vi "Update Impedance.vi"(8 "EEG Data":cluster{"WiBCI16T Data out":T1, "En MAP":u16} {"WiBCI16T Data out"."Reg Map"."ADS2" format="%x"; "WiBCI16T Data out"."Reg Map"."ADS1" format="%x"}, 9 "Numeric":u8, 11 "Data Cluster in":T4) -> (3 "Data Cluster out":T4)   [LabVIEW 2019, in "CML UI.lvlib"]
uses:
  CML UI.lvlib
  Module Data--cluster.ctl
  Acquisition State.ctl
  Measurement UI Displays.ctl
  Acquisition/WiBCI16T_Data.ctl
  Acquisition/WiBCI16T_Status.ctl
  Acquisition/Reg_Map.ctl
  Acquisition/Acquisition.lvlib
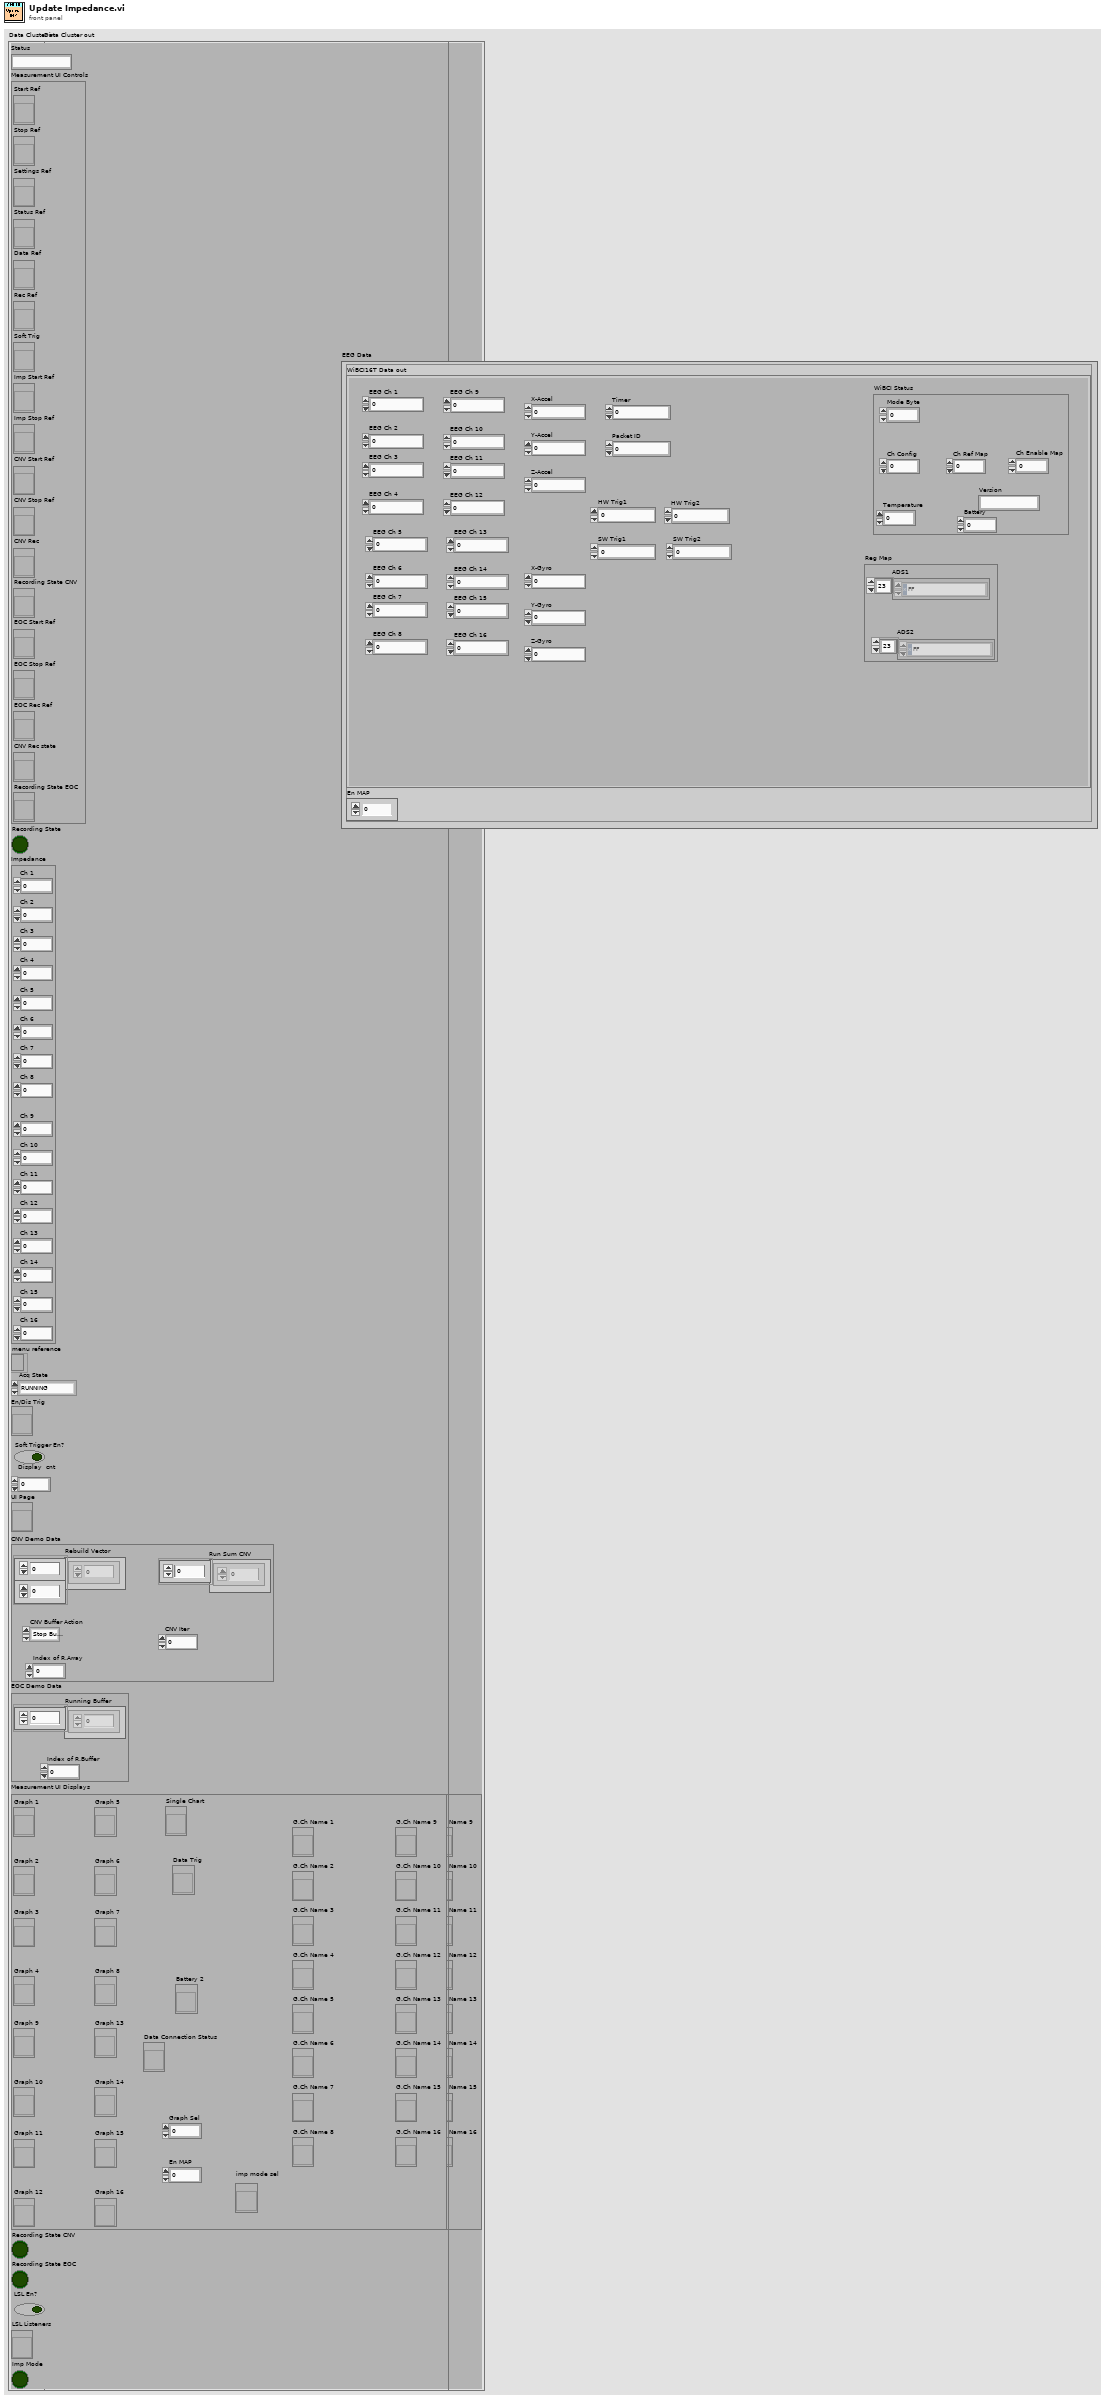
[diagram p1: front panel]
types:
  T1 = typedef "Acquisition.lvlib/WiBCI16T_Data.ctl" = cluster{"EEG Ch 1":dbl, "EEG Ch 2":dbl, "EEG Ch 3":dbl, "EEG Ch 4":dbl, "EEG Ch 5":dbl, "EEG Ch 6":dbl, "EEG Ch 7":dbl, "EEG Ch 8":dbl, "EEG Ch 9":dbl, "EEG Ch 10":dbl, "EEG Ch 11":dbl, "EEG Ch 12":dbl, "EEG Ch 13":dbl, "EEG Ch 14":dbl, "EEG Ch 15":dbl, "EEG Ch 16":dbl, "X-Accel":i16, "Y-Accel":i16, "Z-Accel":i16, "X-Gyro":i16, "Y-Gyro":i16, "Z-Gyro":i16, "Timer":u32, "Packet ID":u32, "HW Trig1":u8, "SW Trig1":i8, "HW Trig2":u8, "SW Trig2":i8, "WiBCI Status":T2, "Reg Map":T3}
  T2 = typedef "Acquisition.lvlib/WiBCI16T_Status.ctl" = cluster{"Mode Byte":u8, "Ch Config":u8, "Ch Ref Map":u16, "Ch Enable Map":u16, "Temperature":sgl, "Battery":u8, "Version":string}
  T3 = typedef "Acquisition.lvlib/Reg_Map.ctl" = cluster{"ADS1":u8[], "ADS2":u8[]}
  T4 = typedef "CML UI.lvlib/Module Data--cluster.ctl" = cluster{"Status":string, "Measurement UI Controls":cluster{"Start Ref":refnum<vi>, "Stop Ref":refnum<vi>, "Settings Ref":refnum<vi>, "Status Ref":refnum<vi>, "Data Ref":refnum<vi>, "Rec Ref":refnum<vi>, "Soft Trig":refnum<vi>, "Imp Start Ref":refnum<vi>, "Imp Stop Ref":refnum<vi>, "CNV Start Ref":refnum<vi>, "CNV Stop Ref":refnum<vi>, "CNV Rec":refnum<vi>, "Recording State CNV":refnum<vi>, "EOC Start Ref":refnum<vi>, "EOC Stop Ref":refnum<vi>, "EOC Rec Ref":refnum<vi>, "CNV Rec state":refnum<vi>, "Recording State EOC":refnum<vi>}, "Recording State":bool, "Impedance":cluster{"Ch 1":dbl, "Ch 2":dbl, "Ch 3":dbl, "Ch 4":dbl, "Ch 5":dbl, "Ch 6":dbl, "Ch 7":dbl, "Ch 8":dbl, "Ch 9":dbl, "Ch 10":dbl, "Ch 11":dbl, "Ch 12":dbl, "Ch 13":dbl, "Ch 14":dbl, "Ch 15":dbl, "Ch 16":dbl}, "menu reference ":refnum<k9>, "Acq State":T5, "En/Dis Trig":refnum<vi>, "Soft Trigger En?":bool, "Display  cnt":u8, "UI Page":refnum<vi>, "CNV Demo Data":cluster{"Rebuild Vector":dbl[][], "CNV Buffer Action":enum16{"Stop Buffer Fill", "Start Buffer Fill", "Analyze Buffer"}, "Index of R.Array":u16, "Run Sum CNV":dbl[], "CNV Iter":u16}, "EOC Demo Data":cluster{"Running Buffer":dbl[], "Index of R.Buffer":u8}, "Measurement UI Displays":T6, "Recording State CNV":bool, "Recording State EOC":bool, "LSL En?":bool, "LSL Listeners":refnum<vi>, "Imp Mode":bool}
  T5 = typedef "CML UI.lvlib/Acquisition State.ctl" = enum16{"RUNNING", "IDLE"}
  T6 = typedef "CML UI.lvlib/Measurement UI Displays.ctl" = cluster{"Graph 1":refnum<vi>, "Graph 2":refnum<vi>, "Graph 3":refnum<vi>, "Graph 4":refnum<vi>, "Graph 5":refnum<vi>, "Graph 6":refnum<vi>, "Graph 7":refnum<vi>, "Graph 8":refnum<vi>, "Graph 9":refnum<vi>, "Graph 10":refnum<vi>, "Graph 11":refnum<vi>, "Graph 12":refnum<vi>, "Graph 13":refnum<vi>, "Graph 14":refnum<vi>, "Graph 15":refnum<vi>, "Graph 16":refnum<vi>, "Battery 2":refnum<vi>, "Data Trig":refnum<vi>, "Data Connection Status":refnum<vi>, "Graph Sel":u8, "En MAP":u16, "Single Chart":refnum<vi>, "G.Ch Name 1":refnum<vi>, "G.Ch Name 2":refnum<vi>, "G.Ch Name 3":refnum<vi>, "G.Ch Name 4":refnum<vi>, "G.Ch Name 5":refnum<vi>, "G.Ch Name 6":refnum<vi>, "G.Ch Name 7":refnum<vi>, "G.Ch Name 8":refnum<vi>, "G.Ch Name 9":refnum<vi>, "G.Ch Name 10":refnum<vi>, "G.Ch Name 11":refnum<vi>, "G.Ch Name 12":refnum<vi>, "G.Ch Name 13":refnum<vi>, "G.Ch Name 14":refnum<vi>, "G.Ch Name 15":refnum<vi>, "G.Ch Name 16":refnum<vi>, "imp mode sel":refnum<vi>}
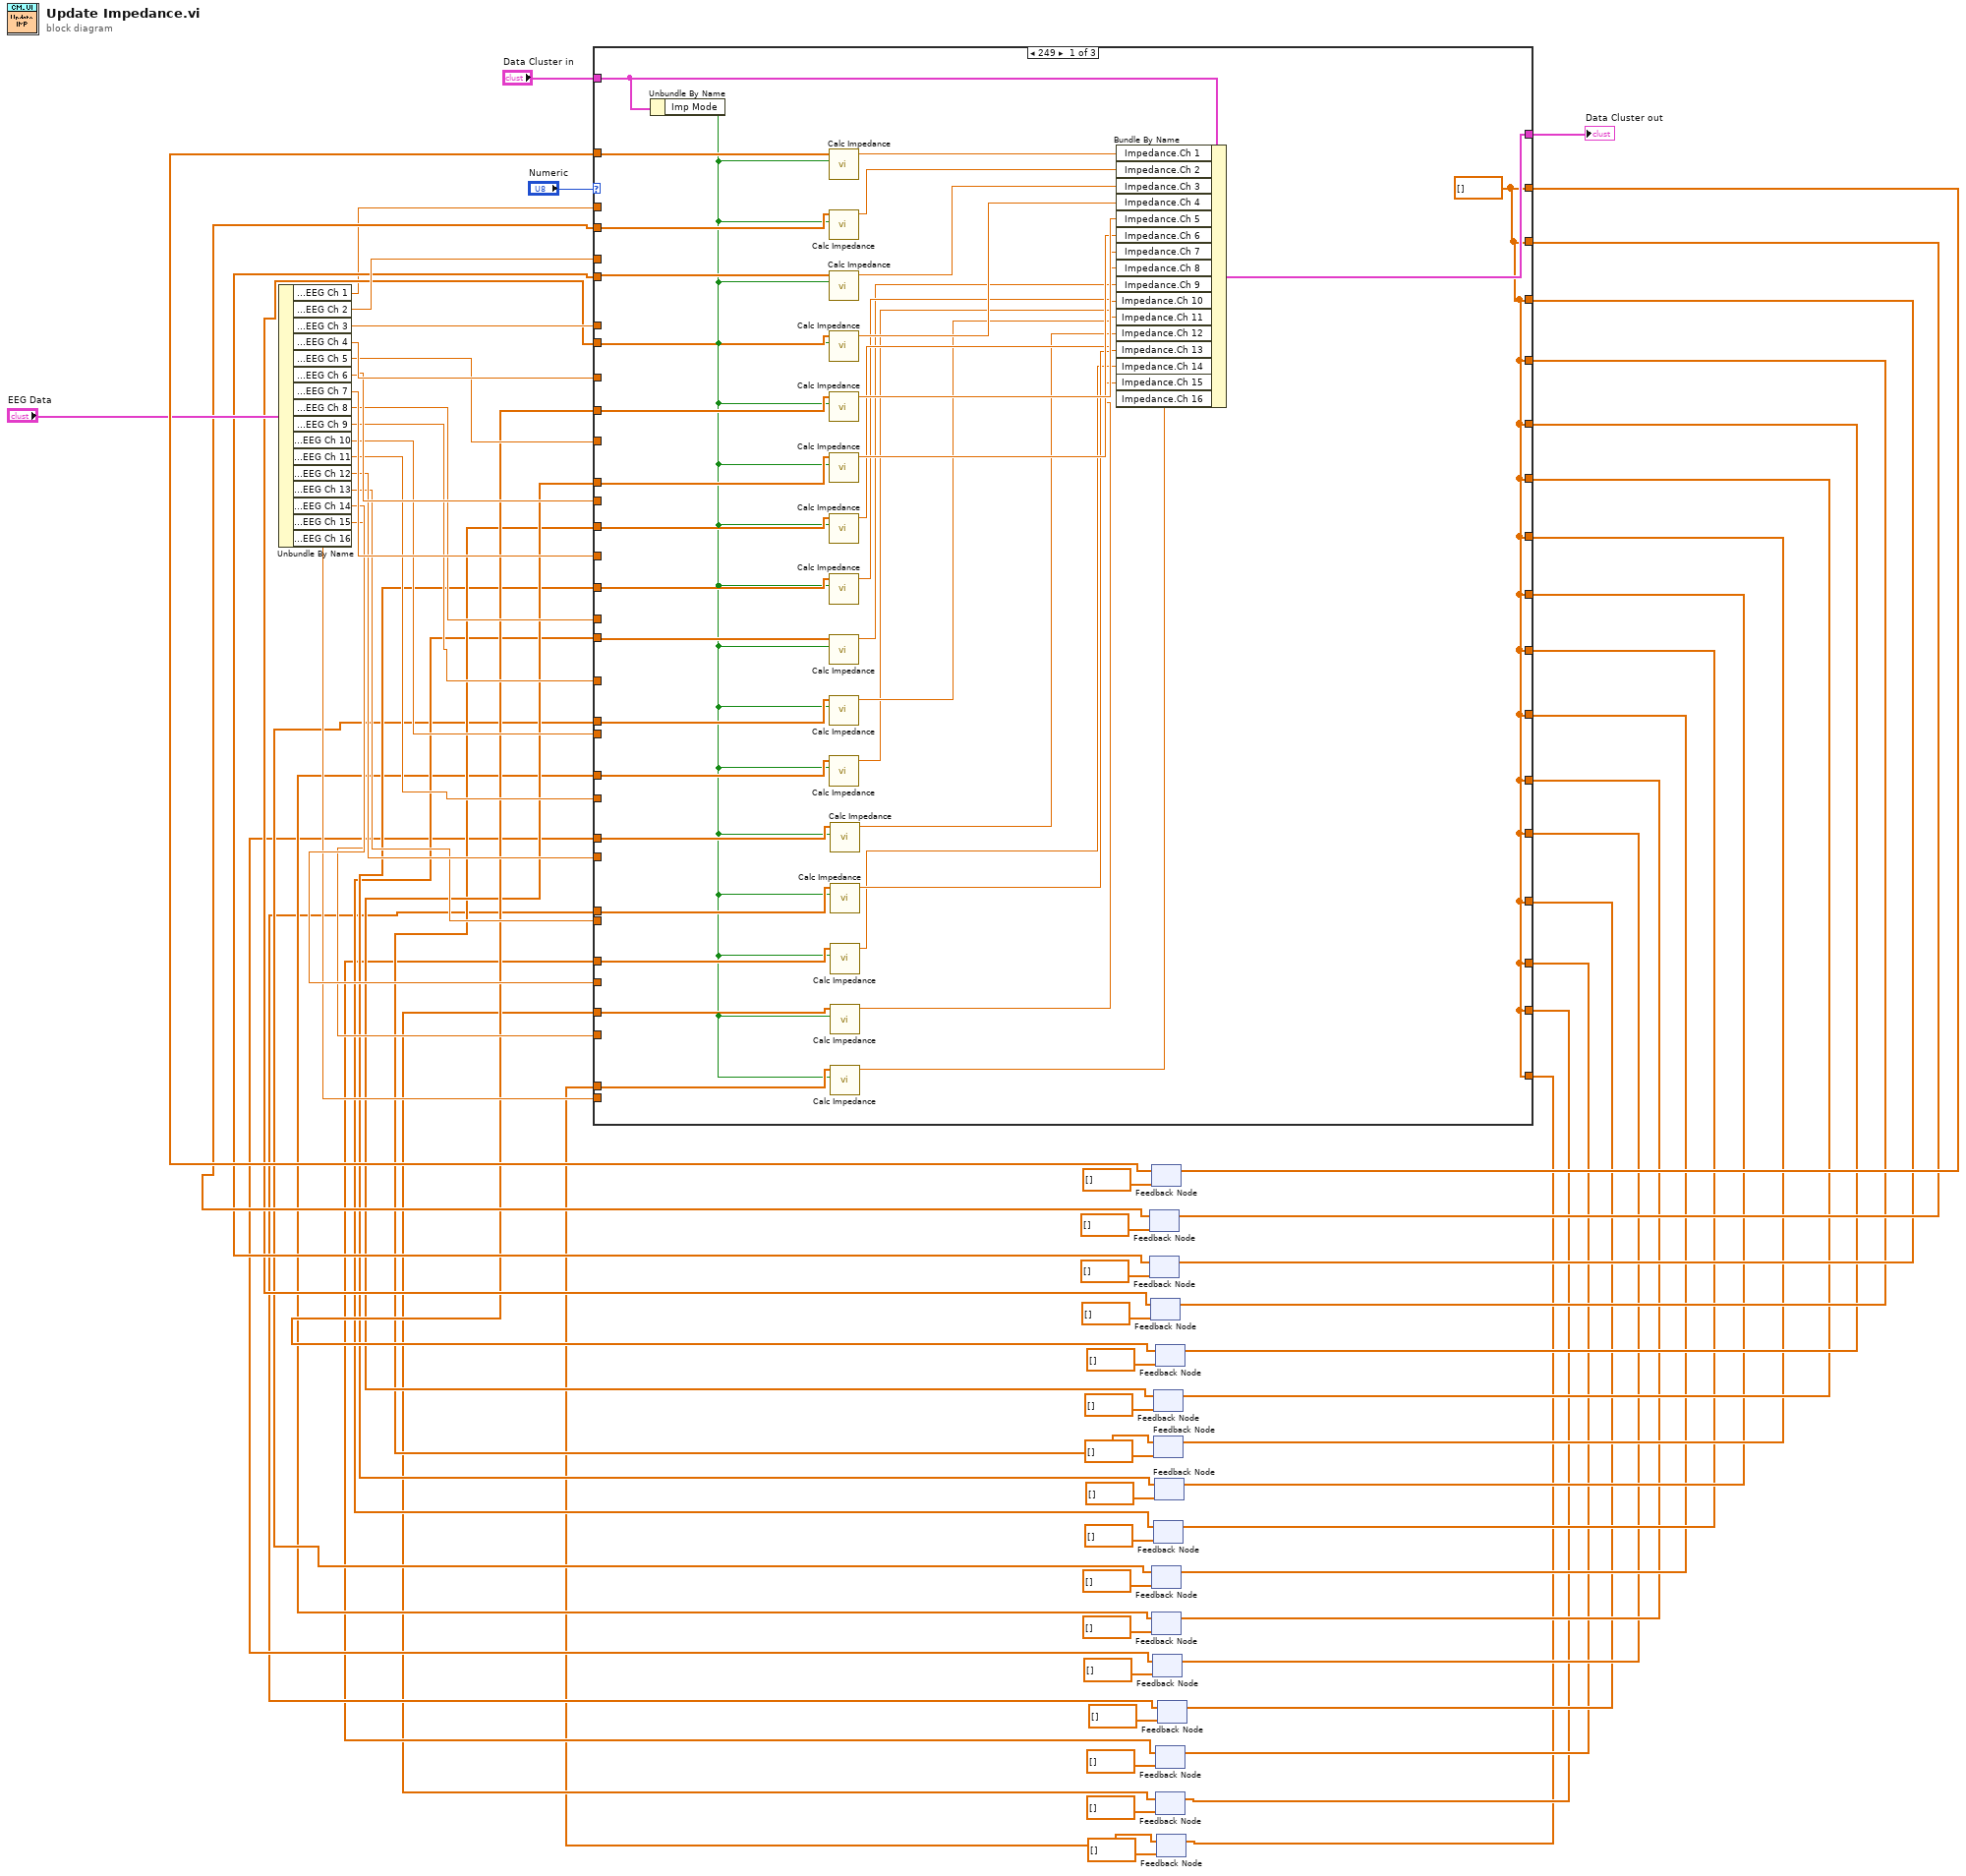
[diagram p0: block diagram]
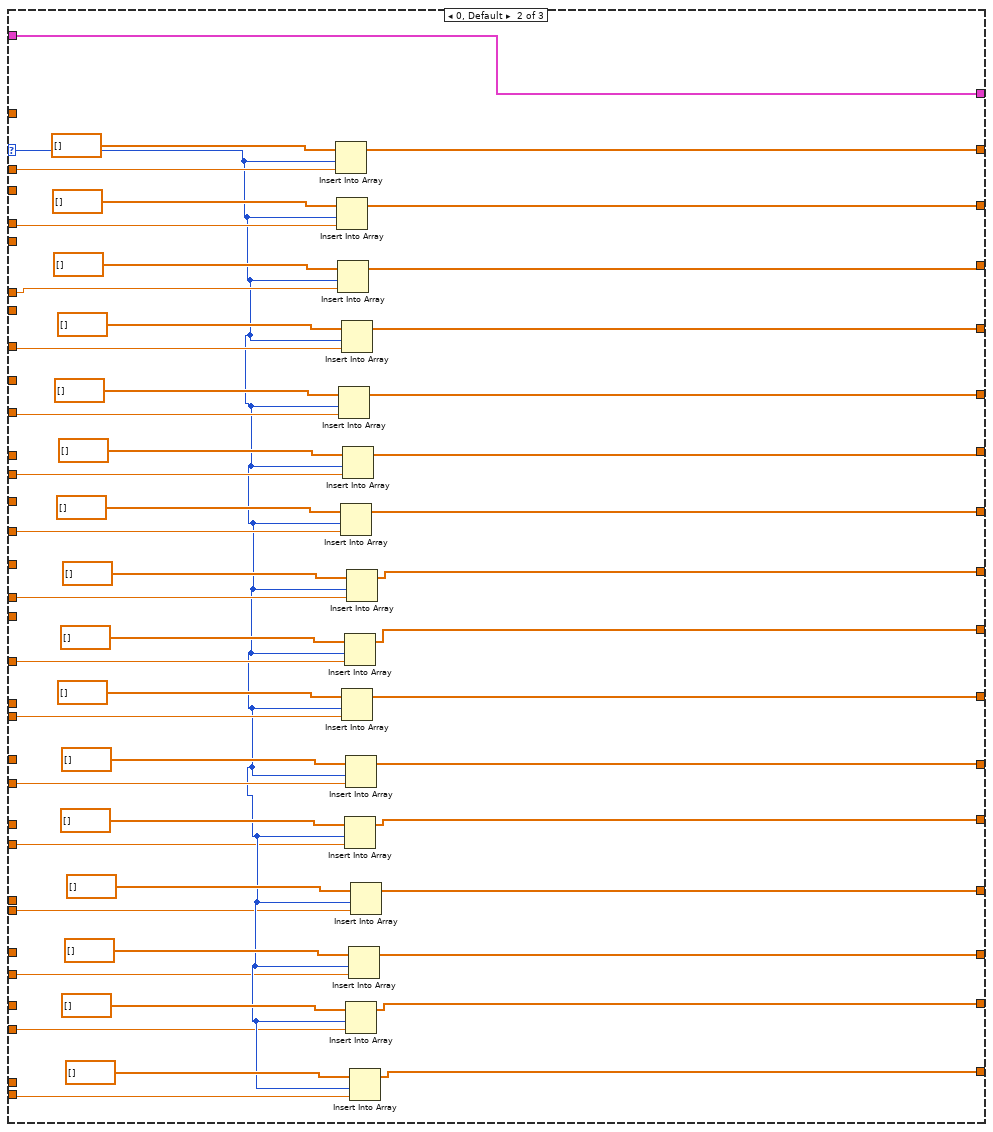
[diagram p2: hidden frame]
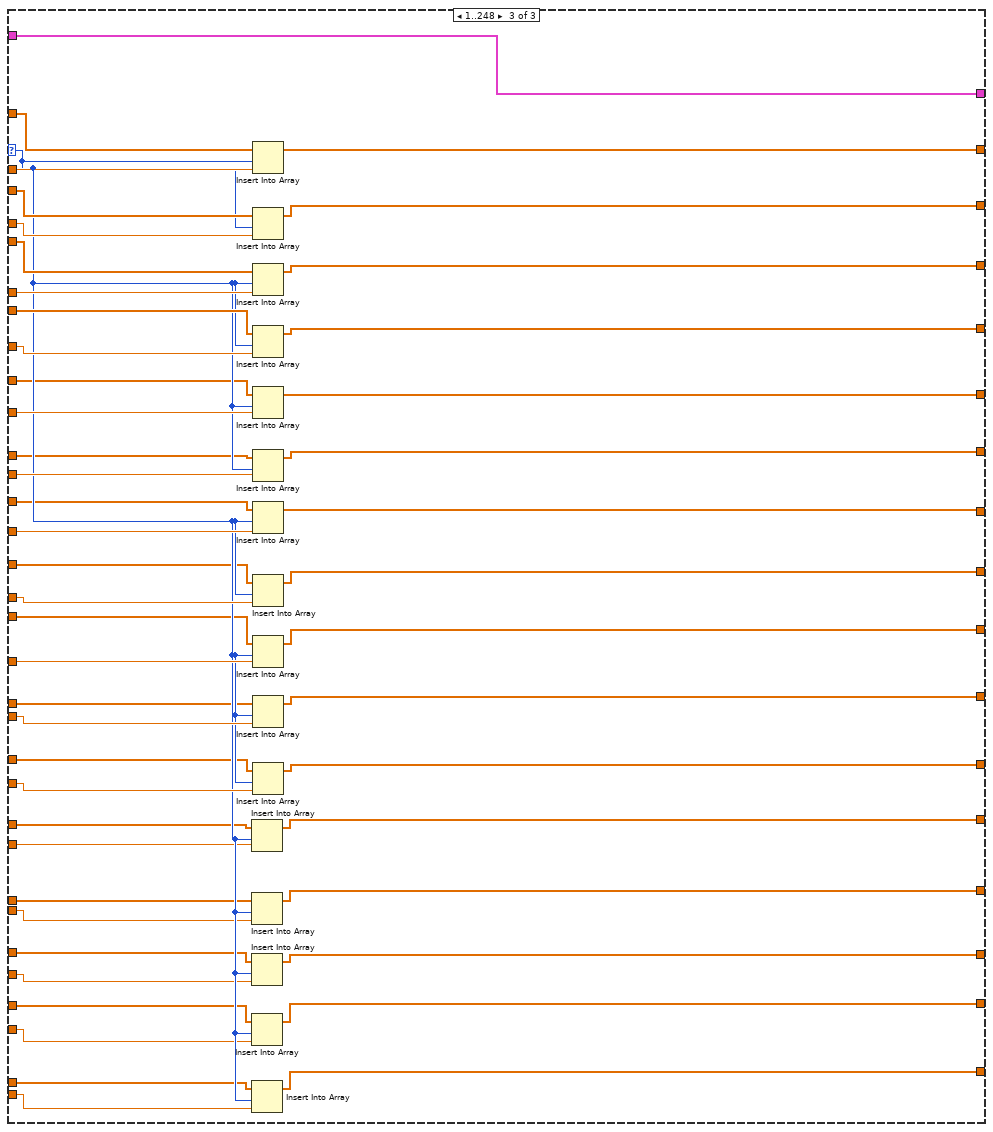
[diagram p3: hidden frame]
diagram:
  n1 = Unbundle By Name("EEG Data") -> ("WiBCI16T Data out.EEG Ch 1"=w1:dbl, "WiBCI16T Data out.EEG Ch 2"=w61:dbl, "WiBCI16T Data out.EEG Ch 3"=w60:dbl, "WiBCI16T Data out.EEG Ch 4"=w59:dbl, "WiBCI16T Data out.EEG Ch 5"=w58:dbl, "WiBCI16T Data out.EEG Ch 6"=w57:dbl, "WiBCI16T Data out.EEG Ch 7"=w56:dbl, "WiBCI16T Data out.EEG Ch 8"=w55:dbl, "WiBCI16T Data out.EEG Ch 9"=w54:dbl, "WiBCI16T Data out.EEG Ch 10"=w53:dbl, "WiBCI16T Data out.EEG Ch 11"=w52:dbl, "WiBCI16T Data out.EEG Ch 12"=w51:dbl, "WiBCI16T Data out.EEG Ch 13"=w50:dbl, "WiBCI16T Data out.EEG Ch 14"=w49:dbl, "WiBCI16T Data out.EEG Ch 15"=w48:dbl, "WiBCI16T Data out.EEG Ch 16"=w47:dbl)
  n2 = feedback #1(dbl[] []) -> (w31:dbl[])
  n3 = feedback #2(dbl[] []) -> (w30:dbl[])
  n4 = feedback #3(dbl[] []) -> (w29:dbl[])
  n5 = feedback #4(dbl[] []) -> (w64:dbl[])
  n6 = feedback #5(dbl[] []) -> (w8:dbl[])
  n7 = feedback #6(dbl[] []) -> (w7:dbl[])
  n8 = feedback #7(dbl[] []) -> (w6:dbl[])
  n9 = feedback #8(dbl[] []) -> (w12:dbl[])
  n10 = feedback #9(dbl[] []) -> (w11:dbl[])
  n11 = feedback #10(dbl[] []) -> (w9:dbl[])
  n12 = feedback #11(dbl[] []) -> (w10:dbl[])
  n13 = feedback #12(dbl[] []) -> (w13:dbl[])
  n14 = feedback #13(dbl[] []) -> (w4:dbl[])
  n15 = feedback #14(dbl[] []) -> (w3:dbl[])
  n16 = feedback #15(dbl[] []) -> (w2:dbl[])
  n17 = feedback #16(dbl[] []) -> (w5:dbl[])
  n18 = case shown="249" "Numeric" {
    selector: "Numeric" -> [_ w125 w177]
    tunnel: [w73 w153 w204] -> w63
    tunnel: w64 -> [w72 _ w202]
    tunnel: w1 -> [_ w152 w203]
    tunnel: "Data Cluster in" -> [w70 w151 w201]
    tunnel: [w103 w151 w201] -> w68
    tunnel: w61 -> [_ w140 w198]
    tunnel: w60 -> [_ w139 w197]
    tunnel: w59 -> [_ w138 w196]
    tunnel: w58 -> [_ w137 w194]
    tunnel: w57 -> [_ w136 w193]
    tunnel: w56 -> [_ w135 w192]
    tunnel: w55 -> [_ w134 w191]
    tunnel: w54 -> [_ w133 w190]
    tunnel: w53 -> [_ w132 w189]
    tunnel: w52 -> [_ w131 w188]
    tunnel: w51 -> [_ w124 w176]
    tunnel: w50 -> [_ w123 w175]
    tunnel: w49 -> [_ w122 w174]
    tunnel: w48 -> [_ w121 w173]
    tunnel: w47 -> [_ w120 w172]
    tunnel: [w73 w119 w187] -> w28
    tunnel: [w73 w118 w186] -> w27
    tunnel: [w73 w117 w185] -> w26
    tunnel: [w73 w116 w184] -> w25
    tunnel: [w73 w115 w183] -> w24
    tunnel: [w73 w114 w182] -> w23
    tunnel: [w73 w113 w181] -> w22
    tunnel: [w73 w112 w180] -> w21
    tunnel: [w73 w111 w179] -> w20
    tunnel: [w73 w110 w178] -> w19
    tunnel: [w73 w109 w171] -> w18
    tunnel: [w73 w108 w170] -> w17
    tunnel: [w73 w107 w169] -> w16
    tunnel: [w73 w106 w168] -> w15
    tunnel: [w73 w105 w167] -> w14
    tunnel: w31 -> [w71 _ w200]
    tunnel: w30 -> [w102 _ w199]
    tunnel: w29 -> [w101 _ w195]
    tunnel: w13 -> [w100 _ w166]
    tunnel: w12 -> [w99 _ w165]
    tunnel: w11 -> [w98 _ w164]
    tunnel: w10 -> [w97 _ w163]
    tunnel: w9 -> [w96 _ w162]
    tunnel: w8 -> [w95 _ w161]
    tunnel: w7 -> [w94 _ w160]
    tunnel: w6 -> [w93 _ w159]
    tunnel: w5 -> [w92 _ w158]
    tunnel: w4 -> [w91 _ w157]
    tunnel: w3 -> [w90 _ w156]
    tunnel: w2 -> [w89 _ w155]
    frame 249 {
      w73 = dbl[] []
      n19 = Unbundle By Name(w70) -> ("Imp Mode"=w69:bool)
      n20 = call "Calc Impedance.vi"("imp mode"=w69, "Array"=w72) -> ("Impedance"=w104:dbl)  [unwired: 9 in]
      n21 = call "Calc Impedance.vi"("imp mode"=w69, "Array"=w71) -> ("Impedance"=w88:dbl)  [unwired: 9 in]
      n22 = call "Calc Impedance.vi"("imp mode"=w69, "Array"=w102) -> ("Impedance"=w87:dbl)  [unwired: 9 in]
      n23 = call "Calc Impedance.vi"("imp mode"=w69, "Array"=w101) -> ("Impedance"=w86:dbl)  [unwired: 9 in]
      n24 = call "Calc Impedance.vi"("imp mode"=w69, "Array"=w100) -> ("Impedance"=w85:dbl)  [unwired: 9 in]
      n25 = call "Calc Impedance.vi"("imp mode"=w69, "Array"=w99) -> ("Impedance"=w84:dbl)  [unwired: 9 in]
      n26 = call "Calc Impedance.vi"("imp mode"=w69, "Array"=w98) -> ("Impedance"=w83:dbl)  [unwired: 9 in]
      n27 = call "Calc Impedance.vi"("imp mode"=w69, "Array"=w97) -> ("Impedance"=w82:dbl)  [unwired: 9 in]
      n28 = call "Calc Impedance.vi"("imp mode"=w69, "Array"=w96) -> ("Impedance"=w81:dbl)  [unwired: 9 in]
      n29 = call "Calc Impedance.vi"("imp mode"=w69, "Array"=w95) -> ("Impedance"=w80:dbl)  [unwired: 9 in]
      n30 = call "Calc Impedance.vi"("imp mode"=w69, "Array"=w94) -> ("Impedance"=w79:dbl)  [unwired: 9 in]
      n31 = call "Calc Impedance.vi"("imp mode"=w69, "Array"=w93) -> ("Impedance"=w78:dbl)  [unwired: 9 in]
      n32 = call "Calc Impedance.vi"("imp mode"=w69, "Array"=w92) -> ("Impedance"=w77:dbl)  [unwired: 9 in]
      n33 = call "Calc Impedance.vi"("imp mode"=w69, "Array"=w91) -> ("Impedance"=w76:dbl)  [unwired: 9 in]
      n34 = call "Calc Impedance.vi"("imp mode"=w69, "Array"=w90) -> ("Impedance"=w75:dbl)  [unwired: 9 in]
      n35 = call "Calc Impedance.vi"("imp mode"=w69, "Array"=w89) -> ("Impedance"=w74:dbl)  [unwired: 9 in]
      n36 = Bundle By Name(cluster=w70, "Impedance.Ch 1"=w104, "Impedance.Ch 2"=w88, "Impedance.Ch 3"=w87, "Impedance.Ch 4"=w86, "Impedance.Ch 5"=w85, "Impedance.Ch 6"=w84, "Impedance.Ch 7"=w83, "Impedance.Ch 8"=w82, "Impedance.Ch 9"=w81, "Impedance.Ch 10"=w80, "Impedance.Ch 11"=w79, "Impedance.Ch 12"=w78, "Impedance.Ch 13"=w77, "Impedance.Ch 14"=w76, "Impedance.Ch 15"=w75, "Impedance.Ch 16"=w74) -> (w103:T4)
    }
    frame 0, Default {
      n37 = Insert Into Array(array=dbl[] [], index=w125, new element=w152) -> (w153:dbl[])
      n38 = Insert Into Array(array=dbl[] [], index=w125, new element=w140) -> (w119:dbl[])
      n39 = Insert Into Array(array=dbl[] [], index=w125, new element=w139) -> (w118:dbl[])
      n40 = Insert Into Array(array=dbl[] [], index=w125, new element=w137) -> (w116:dbl[])
      n41 = Insert Into Array(array=dbl[] [], index=w125, new element=w135) -> (w114:dbl[])
      n42 = Insert Into Array(array=dbl[] [], index=w125, new element=w138) -> (w117:dbl[])
      n43 = Insert Into Array(array=dbl[] [], index=w125, new element=w132) -> (w111:dbl[])
      n44 = Insert Into Array(array=dbl[] [], index=w125, new element=w136) -> (w115:dbl[])
      n45 = Insert Into Array(array=dbl[] [], index=w125, new element=w133) -> (w112:dbl[])
      n46 = Insert Into Array(array=dbl[] [], index=w125, new element=w124) -> (w109:dbl[])
      n47 = Insert Into Array(array=dbl[] [], index=w125, new element=w131) -> (w110:dbl[])
      n48 = Insert Into Array(array=dbl[] [], index=w125, new element=w121) -> (w106:dbl[])
      n49 = Insert Into Array(array=dbl[] [], index=w125, new element=w134) -> (w113:dbl[])
      n50 = Insert Into Array(array=dbl[] [], index=w125, new element=w122) -> (w107:dbl[])
      n51 = Insert Into Array(array=dbl[] [], index=w125, new element=w120) -> (w105:dbl[])
      n52 = Insert Into Array(array=dbl[] [], index=w125, new element=w123) -> (w108:dbl[])
    }
    frame 1..248 {
      n53 = Insert Into Array(array=w159, index=w177, new element=w176) -> (w171:dbl[])
      n54 = Insert Into Array(array=w158, index=w177, new element=w175) -> (w170:dbl[])
      n55 = Insert Into Array(array=w157, index=w177, new element=w174) -> (w169:dbl[])
      n56 = Insert Into Array(array=w156, index=w177, new element=w173) -> (w168:dbl[])
      n57 = Insert Into Array(array=w155, index=w177, new element=w172) -> (w167:dbl[])
      n58 = Insert Into Array(array=w202, index=w177, new element=w203) -> (w204:dbl[])
      n59 = Insert Into Array(array=w200, index=w177, new element=w198) -> (w187:dbl[])
      n60 = Insert Into Array(array=w199, index=w177, new element=w197) -> (w186:dbl[])
      n61 = Insert Into Array(array=w195, index=w177, new element=w196) -> (w185:dbl[])
      n62 = Insert Into Array(array=w166, index=w177, new element=w194) -> (w184:dbl[])
      n63 = Insert Into Array(array=w165, index=w177, new element=w193) -> (w183:dbl[])
      n64 = Insert Into Array(array=w164, index=w177, new element=w192) -> (w182:dbl[])
      n65 = Insert Into Array(array=w163, index=w177, new element=w191) -> (w181:dbl[])
      n66 = Insert Into Array(array=w162, index=w177, new element=w190) -> (w180:dbl[])
      n67 = Insert Into Array(array=w161, index=w177, new element=w189) -> (w179:dbl[])
      n68 = Insert Into Array(array=w160, index=w177, new element=w188) -> (w178:dbl[])
    }
  }
  "Data Cluster out" <- w68
  n69 = feedback-in #1(w28) -> ()
  n70 = feedback-in #2(w27) -> ()
  n71 = feedback-in #3(w26) -> ()
  n72 = feedback-in #4(w63) -> ()
  n73 = feedback-in #5(w20) -> ()
  n74 = feedback-in #6(w19) -> ()
  n75 = feedback-in #7(w18) -> ()
  n76 = feedback-in #8(w24) -> ()
  n77 = feedback-in #9(w23) -> ()
  n78 = feedback-in #10(w21) -> ()
  n79 = feedback-in #11(w22) -> ()
  n80 = feedback-in #12(w25) -> ()
  n81 = feedback-in #13(w16) -> ()
  n82 = feedback-in #14(w15) -> ()
  n83 = feedback-in #15(w14) -> ()
  n84 = feedback-in #16(w17) -> ()
